vi "GetXArray.vi"(8 "error in (no error)":errorcluster, 9 "TraceID":i32, 10 "GraphID":i32, 11 "VISA resource name":refnum<visa-resource-name>) -> (0 "error out":errorcluster, 2 "xArray":string, 3 "VISA resource name out":refnum<visa-resource-name>)   [LabVIEW 2014, in "Stanford Research SR1.lvlib"]
doc: "Reads out the x array of a specific trace."
uses:
  Stanford Research SR1.lvlib
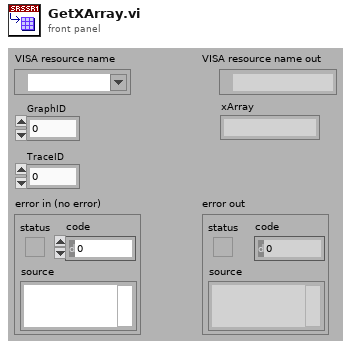
[diagram p1: front panel]
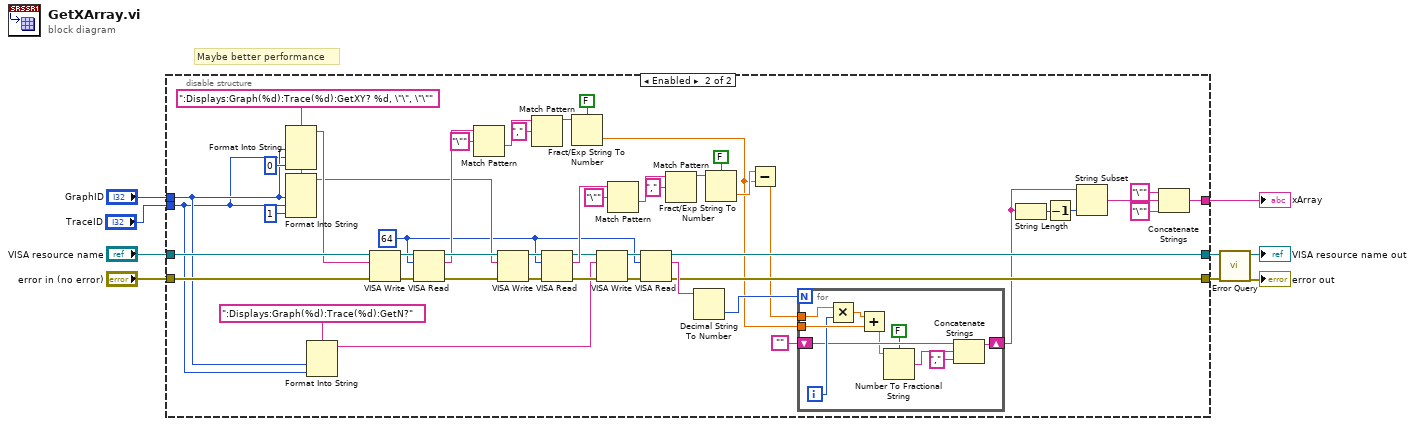
[diagram p0: block diagram]
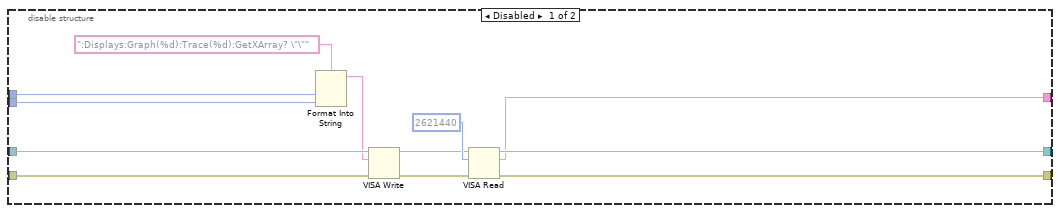
[diagram p2: hidden frame]
diagram:
  # "Maybe better performance"
  n1 = disable-structure shown="Enabled" {
    disable-tunnel: "VISA resource name" -> [w21 w64]
    disable-tunnel: "error in (no error)" -> [w20 w63]
    disable-tunnel: [w16 w33] -> w7
    disable-tunnel: [w15 w34] -> w6
    disable-tunnel: "GraphID" -> [w13 w41]
    disable-tunnel: "TraceID" -> [w11 w40]
    disable-tunnel: [w10 w24] -> w1
    frame Disabled {
      n2 = Format Into String(format string=":Displays:Graph(%d):Trace(%d):GetXArray? \"\"", w13, w11) -> (resulting string=w12:string)  [unwired: 2 in, 1 out]
      n3 = VISA Write(VISA resource name=w21, write buffer=w12, error in (no error)=w20) -> (VISA resource name out=w18:refnum<visa-resource-name>, error out=w17:errorcluster)  [unwired: 1 out]
      n4 = VISA Read(VISA resource name=w18, byte count=2621440, error in (no error)=w17) -> (VISA resource name out=w16:refnum<visa-resource-name>, read buffer=w10:string, error out=w15:errorcluster)  [unwired: 1 out]
    }
    frame Enabled {
      w50 = ":Displays:Graph(%d):Trace(%d):GetXY? %d, \"\", \"\"" ("format string")
      w36 = 64
      n5 = Format Into String(format string=w50, w41, w40, 0 ("input 3")) -> (resulting string=w49:string)  [unwired: 2 in, 1 out]
      n6 = Format Into String(format string=w50, w41, w40, 1 ("input 3")) -> (resulting string=w48:string)  [unwired: 2 in, 1 out]
      n7 = Format Into String(format string=":Displays:Graph(%d):Trace(%d):GetN?", w41, w40) -> (resulting string=w38:string)  [unwired: 2 in, 1 out]
      n8 = VISA Write(VISA resource name=w64, write buffer=w49, error in (no error)=w63) -> (VISA resource name out=w69:refnum<visa-resource-name>, error out=w70:errorcluster)  [unwired: 1 out]
      n9 = VISA Read(VISA resource name=w69, byte count=w36, error in (no error)=w70) -> (VISA resource name out=w65:refnum<visa-resource-name>, read buffer=w57:string, error out=w66:errorcluster)  [unwired: 1 out]
      n10 = Match Pattern(string=w57, regular expression="\"") -> (after substring=w61:string)  [unwired: 1 in, 3 out]
      n11 = VISA Write(VISA resource name=w65, write buffer=w48, error in (no error)=w66) -> (VISA resource name out=w68:refnum<visa-resource-name>, error out=w67:errorcluster)  [unwired: 1 out]
      n12 = Match Pattern(string=w61, regular expression=",") -> (before substring=w59:string)  [unwired: 1 in, 3 out]
      n13 = VISA Read(VISA resource name=w68, byte count=w36, error in (no error)=w67) -> (VISA resource name out=w42:refnum<visa-resource-name>, read buffer=w51:string, error out=w43:errorcluster)  [unwired: 1 out]
      n14 = Fract/Exp String To Number(use system decimal point (T)=FALSE, string=w59) -> (number=w30:dbl)  [unwired: 2 in, 1 out]
      n15 = VISA Write(VISA resource name=w42, write buffer=w38, error in (no error)=w43) -> (VISA resource name out=w44:refnum<visa-resource-name>, error out=w45:errorcluster)  [unwired: 1 out]
      n16 = Match Pattern(string=w51, regular expression="\"") -> (after substring=w55:string)  [unwired: 1 in, 3 out]
      n17 = VISA Read(VISA resource name=w44, byte count=w36, error in (no error)=w45) -> (VISA resource name out=w33:refnum<visa-resource-name>, read buffer=w37:string, error out=w34:errorcluster)  [unwired: 1 out]
      n18 = Match Pattern(string=w55, regular expression=",") -> (before substring=w53:string)  [unwired: 1 in, 3 out]
      n19 = Decimal String To Number(string=w37) -> (number=w35:i32)  [unwired: 2 in, 1 out]
      n20 = Fract/Exp String To Number(use system decimal point (T)=FALSE, string=w53) -> (number=w32:dbl)  [unwired: 2 in, 1 out]
      n21 = Subtract(x=w32, y=w30) -> (x-y=w31:dbl)
      n22 = for {
        N: w35 -> [_]
        tunnel: w31 -> [w78]
        shift-right: [w76] -> w28
        shift-left: "" -> [w75]
        tunnel: w30 -> [w80]
        i -> [w77]
        n23 = Multiply(x=w78, y=w77) -> (x*y=w79:dbl)
        n24 = Add(x=w79, y=w80) -> (x+y=w73:dbl)
        n25 = Number To Fractional String(use system decimal point (T)=FALSE, number=w73) -> (F-format string=w74:string)  [unwired: 2 in]
        n26 = Concatenate Strings(w75, w74, "," ("string")) -> (w76:string)
      }
      n27 = String Length(string=w28) -> (length=w27:i32)
      n28 = Decrement(x=w27) -> (x-1=w26:i32)
      n29 = String Subset(string=w28, length (rest)=w26) -> (substring=w25:string)  [unwired: 1 in]
      n30 = Concatenate Strings("\"" ("string"), w25, "\"" ("string")) -> (w24:string)
    }
  }
  "xArray" <- w1
  n31 = call "Error Query.vi"("error in (no error)"=w6, "VISA resource name"=w7) -> ("error out"=→"error out":errorcluster, "VISA resource name out"=→"VISA resource name out":refnum<visa-resource-name>)  [unwired: 6 in, 2 out]
